vi "Dual State Press Change.vi"(1 "Enable/Disable":bool) -> (0 "Enabled":bool)   [LabVIEW 2011]
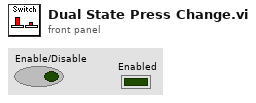
[diagram p1: front panel]
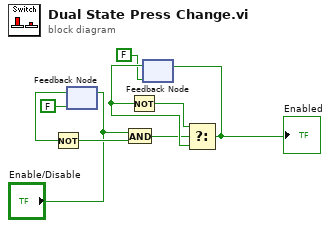
[diagram p0: block diagram]
diagram:
  n1 = feedback #1(FALSE ("Button 3")) -> (w2:bool)
  n2 = Not(x=w2) -> (.not. x?=w3:bool)
  n3 = feedback-in #1("Enable/Disable") -> ()
  n4 = And(x="Enable/Disable", y=w3) -> (x .and. y?=w6:bool)
  n5 = feedback #2(FALSE) -> (w8:bool)
  n6 = Not(x=w8) -> (.not. x?=w7:bool)
  n7 = Select(t=w7, s=w6, f=w8) -> (s? t:f=w9:bool)
  "Enabled" <- w9
  n8 = feedback-in #2(w9) -> ()
